vi "VciDeviceOpen.vi"(3 "error in":errorcluster {"code" format="%.0x"}, 5 "Device ID":cluster{"Low Part":u32, "High Part":u32} {"High Part" format="%08x"; "Low Part" format="%08x"}) -> (0 "error out":errorcluster {"code" format="%.0x"}, 2 "Device Handle":u32 format="%x")   [LabVIEW 2011]
doc: "Opens the VCI device specified by Device ID."
uses:
  vcilva.dll
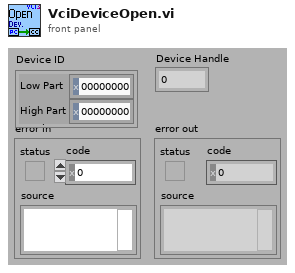
[diagram p1: front panel]
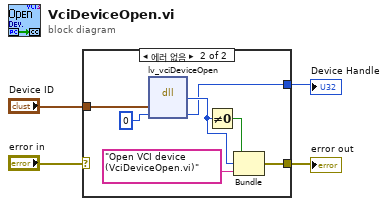
[diagram p0: block diagram]
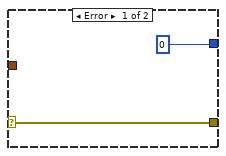
[diagram p2: hidden frame]
diagram:
  n1 = case shown="에러 없음" "error in" {
    selector: "error in" -> [w6 _]
    tunnel: [w6 w13] -> w3
    tunnel: "Device ID" -> [_ w9]
    tunnel: [0 w8] -> w1
    frame Error {
    }
    frame No Error {
      n2 = dll-call lib="vcilva.dll" fn="lv_vciDeviceOpen"("Device ID"=w9, "hDevice"=u32 0) -> (w10:i32, "hDevice"=w8:u32)  [unwired: 4 in, 2 out]
      n3 = Not Equal To 0?(x=w10) -> (x != 0?=w12:bool)
      n4 = Bundle(w12, w10, "Open VCI device (VciDeviceOpen.vi)") -> (w13:errorcluster)  [unwired: 1 in]
    }
  }
  "error out" <- w3
  "Device Handle" <- w1
